vi "String to dbl1.vi"(11 "String":string) -> (2 "Error?":bool, 3 "dbl":dbl)   [LabVIEW 2018, in "Main.lvlib"]
uses:
  Main.lvlib
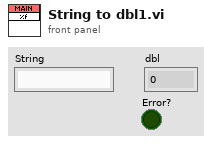
[diagram p1: front panel]
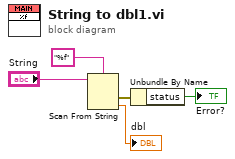
[diagram p0: block diagram]
diagram:
  n1 = Scan From String(format string="%f", input string="String") -> (error out=w2:errorcluster, output 1=→"dbl":dbl)  [unwired: 3 in, 2 out]
  n2 = Unbundle By Name(w2) -> ("status"=→"Error?":bool)
